vi "atMonochromator_logEvent_LightStatus.vi"(8 "error in (no error)":errorcluster, 11 "logevent_LightStatus_Ctl":T1) -> (0 "error out":errorcluster, 2 "function return":i32, 3 "logevent_LightStatus_Ctl out":T1)   [LabVIEW 2016, in "SALLV_atMonochromator.lvlib"]
doc: "int atMonochromator_shm_logEvent_LightStatusLV(atMonochromator_logevent_LightStatusLV *logevent_LightStatus_Ctl );"
uses:
  SALLV_atMonochromator.lvlib
  DataTypes/logevent_LightStatus.ctl
  SALLV_atMonochromator.so
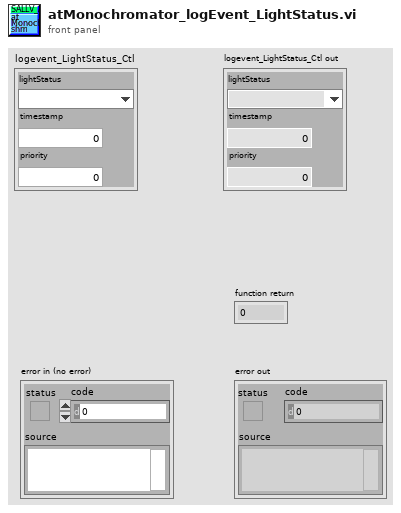
[diagram p1: front panel]
types:
  T1 = typedef "SALLV_atMonochromator.lvlib/logevent_LightStatus.ctl" = cluster{"lightStatus":enum16{"", "On", "Off"}, "timestamp":dbl, "priority":i32}
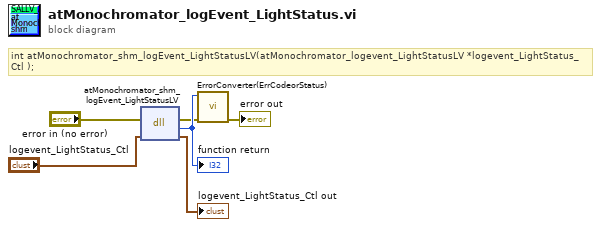
[diagram p0: block diagram]
diagram:
  # "int atMonochromator_shm_logEvent_LightStatusLV(atMonochromator_logevent_LightStatusLV *logevent_LightStatus_Ctl );"
  n1 = dll-call lib="home/andres/Desktop/SAL_atMonochromator/SALLV_atMonochromator.*" fn="atMonochromator_shm_logEvent_LightStatusLV"(error in="error in (no error)", "logevent_LightStatus_Ctl"="logevent_LightStatus_Ctl") -> (error out=w2:errorcluster, w6:i32, "logevent_LightStatus_Ctl"=→"logevent_LightStatus_Ctl out":T1)  [unwired: 2 in, 1 out]
  "function return" <- w6
  n2 = call "ErrorConverter(ErrCodeorStatus).vi"("error in (no error)"=w2, "error code"=w6) -> ("error out"=→"error out":errorcluster)  [unwired: 9 in]
